vi "标样核查.vi"(11 "标样核查配置":T1={"数据保存间隔"=1.0, "水温标样值"=0.0, "pH标样值"=0.0, "溶解氧标样值"=0.0, "电导率标样值"=0.0, "浊度标样值"=0.0}) -> ()   [LabVIEW 2016, in "斯坦道多参数.lvlib"]
panel:
  out "运行状态":u16(ring) items=["空闲", "水样测试", "标样核查"]
  out "seconds since 1Jan1904":timestamp
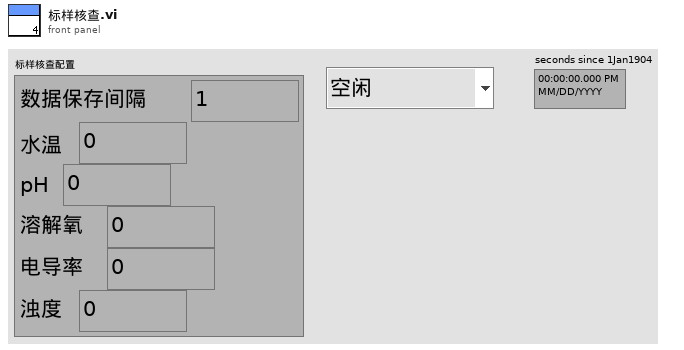
[diagram p1: front panel]
types:
  T1 = cluster{"数据保存间隔":dbl, "水温标样值":dbl, "pH标样值":dbl, "溶解氧标样值":dbl, "电导率标样值":dbl, "浊度标样值":dbl}
  T2 = cluster{"因子编码":string, "单位":string, "标样参考值":sgl, "水样数据时间":timestamp, "水样实测值":sgl, "水样数据标识":string, "探头温度":sgl}
  T3 = typedef "LVDateTimeRec.ctl" = cluster{"秒数的小数部分":dbl, "秒":i32, "分":i32, "时":i32, "日":i32, "月":i32, "年":i32, "天数（周）":i32, "天数（年）":i32, "DST":i32}
  T4 = cluster{"温度测量值":sgl, "DO%":sgl, "DOmg/L":sgl, "温度偏移修正值":sgl}
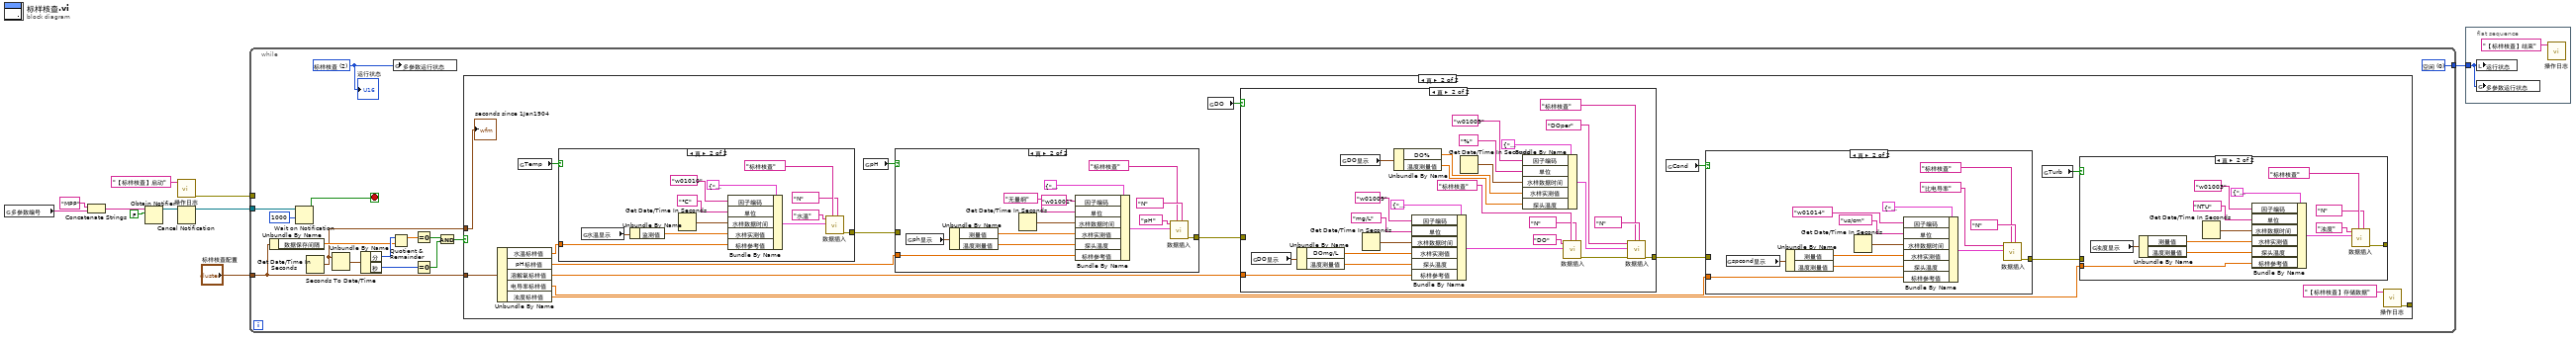
[diagram p0: block diagram]
diagram:
  n1 = global read "多参数全局变量.vi" "多参数编号"() -> (w3:string)
  n2 = Concatenate Strings("MPP" ("名称（未命名）"), w3) -> (w4:string)
  n3 = Obtain Notifier(name (unnamed)=w4, notification data type=FALSE) -> (notifier out=w7:refnum<notifier>)  [unwired: 2 in, 2 out]
  n4 = call "操作日志.vi"("日志信息"="【标样核查】启动") -> ("error out"=w1:errorcluster)  [unwired: 10 in]
  n5 = Cancel Notification(0:w7) -> (8:w6:refnum<notifier>)  [unwired: 1 in, 2 out]
  n6 = while {
    tunnel: "标样核查配置" -> [w21]
    tunnel: [w15] -> w5
    tunnel: w6 -> [w14]
    tunnel: w1 -> [_]
    stop <- w12 stop-if-true
    w15 = u16 0 items=["空闲", "水样测试", "标样核查"] ("多参数运行状态")
    w11 = u16 2 items=["空闲", "水样测试", "标样核查"] ("多参数运行状态")
    n7 = Unbundle By Name(w21) -> ("数据保存间隔"=w19:dbl)
    n8 = Wait on Notification(notifier=w14, timeout in ms (-1)=1000 ("超时毫秒(-1)")) -> (notification=w12:bool)  [unwired: 2 in, 3 out]
    n9 = Get Date/Time In Seconds() -> (seconds since 1Jan1904=w16:timestamp)
    n10 = Seconds To Date/Time(time stamp (now)=w16) -> (date time rec=w25:T3)  [unwired: 1 in]
    n11 = Unbundle By Name(w25) -> ("分"=w20:i32, "秒"=w24:i32)
    n12 = Quotient & Remainder(x=w20, y=w19) -> (x-y*floor(x/y)=w18:dbl)  [unwired: 1 out]
    n13 = global write "多参数全局变量.vi" "多参数运行状态"(w11) -> ()
    n14 = Equal To 0?(x=w18) -> (x = 0?=w17:bool)
    n15 = Equal To 0?(x=w24) -> (x = 0?=w23:bool)
    n16 = And(x=w17, y=w23) -> (x .and. y?=w22:bool)
    n17 = case shown="真" w22 {
      tunnel: w21 -> [_ w33]
      tunnel: w16 -> [_ w43]
      tunnel: [_ w26] -> _
      frame False {
      }
      frame True {
        n18 = Unbundle By Name(w33) -> ("水温标样值"=w32:dbl, "pH标样值"=w31:dbl, "溶解氧标样值"=w30:dbl, "电导率标样值"=w29:dbl, "浊度标样值"=w28:dbl)
        n19 = global read "断电保存变量.vi" "Temp"() -> (w38:bool)
        n20 = case shown="真" w38 {
          tunnel: [_ w111] -> w42
          tunnel: w32 -> [_ w110]
          frame False {
          }
          frame True {
            n21 = global read "多参数全局变量.vi" "水温显示"() -> (w109:cluster{"CH":u16, "监测值":dbl, "温度偏移修正值":sgl})
            n22 = Unbundle By Name(w109) -> ("监测值"=w108:dbl)
            n23 = Get Date/Time In Seconds() -> (seconds since 1Jan1904=w118:timestamp)
            n24 = Bundle By Name(cluster=T2 {"因子编码"="w01003", "单位"="无量纲", "标样参考值"=0.0, "水样数据时间"=timestamp(0 s since 1904-01-01), "水样实测值"=0.0, "水样数据标识"="N", "探头温度"=0.0} ("data in"), "因子编码"="w01010", "单位"="℃", "水样数据时间"=w118, "水样实测值"=w108, "标样参考值"=w110) -> (w117:T2)
            n25 = call "数据插入.vi"("数据标记表"="N", "测量模式"="标样核查", "data in"=w117, "table输入"="水温") -> ("error out"=w111:errorcluster)  [unwired: 7 in]
          }
        }
        n26 = global read "断电保存变量.vi" "pH"() -> (w37:bool)
        n27 = case shown="真" w37 {
          tunnel: w42 -> [_ _]
          tunnel: [_ w99] -> w41
          tunnel: w31 -> [_ w98]
          frame False {
          }
          frame True {
            n28 = global read "多参数全局变量.vi" "ph显示"() -> (w97:cluster{"温度测量值":sgl, "测量值":sgl, "温度偏移修正值":sgl})
            n29 = Unbundle By Name(w97) -> ("测量值"=w96:sgl, "温度测量值"=w95:sgl)
            n30 = Get Date/Time In Seconds() -> (seconds since 1Jan1904=w104:timestamp)
            n31 = Bundle By Name(cluster=T2 {"因子编码"="w01003", "单位"="无量纲", "标样参考值"=0.0, "水样数据时间"=timestamp(0 s since 1904-01-01), "水样实测值"=0.0, "水样数据标识"="N", "探头温度"=0.0} ("data in"), "因子编码"="w01001", "单位"="无量纲", "水样数据时间"=w104, "水样实测值"=w96, "探头温度"=w95, "标样参考值"=w98) -> (w105:T2)
            n32 = call "数据插入.vi"("数据标记表"="N", "测量模式"="标样核查", "data in"=w105, "table输入"="pH") -> ("error out"=w99:errorcluster)  [unwired: 7 in]
          }
        }
        n33 = global read "断电保存变量.vi" "DO"() -> (w36:bool)
        n34 = case shown="真" w36 {
          tunnel: w41 -> [_ _]
          tunnel: [_ w82] -> w40
          tunnel: w30 -> [_ w84]
          frame False {
          }
          frame True {
            n35 = global read "多参数全局变量.vi" "DO显示"() -> (w70:T4)
            n36 = Unbundle By Name(w70) -> ("DOmg/L"=w92:sgl, "温度测量值"=w94:sgl)
            n37 = global read "多参数全局变量.vi" "DO显示"() -> (w71:T4)
            n38 = Get Date/Time In Seconds() -> (seconds since 1Jan1904=w91:timestamp)
            n39 = Unbundle By Name(w71) -> ("DO%"=w75:sgl, "温度测量值"=w73:sgl)
            n40 = Bundle By Name(cluster=T2 {"因子编码"="w01003", "单位"="无量纲", "标样参考值"=0.0, "水样数据时间"=timestamp(0 s since 1904-01-01), "水样实测值"=0.0, "水样数据标识"="N", "探头温度"=0.0} ("data in"), "因子编码"="w01009", "单位"="mg/L", "水样数据时间"=w91, "水样实测值"=w92, "探头温度"=w94, "标样参考值"=w84) -> (w90:T2)
            n41 = Get Date/Time In Seconds() -> (seconds since 1Jan1904=w76:timestamp)
            n42 = Bundle By Name(cluster=T2 {"因子编码"="w01003", "单位"="无量纲", "标样参考值"=0.0, "水样数据时间"=timestamp(0 s since 1904-01-01), "水样实测值"=0.0, "水样数据标识"="N", "探头温度"=0.0} ("data in"), "因子编码"="w01009", "单位"="%", "水样数据时间"=w76, "水样实测值"=w75, "探头温度"=w73) -> (w72:T2)
            n43 = call "数据插入.vi"("数据标记表"="N", "测量模式"="标样核查", "data in"=w90, "table输入"="DO") -> ("error out"=w83:errorcluster)  [unwired: 7 in]
            n44 = call "数据插入.vi"("数据标记表"="N", "测量模式"="标样核查", "error in (no error)"=w83, "data in"=w72, "table输入"="DOper") -> ("error out"=w82:errorcluster)  [unwired: 6 in]
          }
        }
        n45 = global read "断电保存变量.vi" "Cond"() -> (w35:bool)
        n46 = case shown="真" w35 {
          tunnel: w40 -> [_ _]
          tunnel: [_ w61] -> w39
          tunnel: w29 -> [_ w60]
          frame False {
          }
          frame True {
            n47 = global read "多参数全局变量.vi" "spcond显示"() -> (w59:cluster{"温度测量值":sgl, "测量值":sgl, "温度偏移修正值":sgl})
            n48 = Unbundle By Name(w59) -> ("测量值"=w58:sgl, "温度测量值"=w57:sgl)
            n49 = Get Date/Time In Seconds() -> (seconds since 1Jan1904=w66:timestamp)
            n50 = Bundle By Name(cluster=T2 {"因子编码"="w01003", "单位"="无量纲", "标样参考值"=0.0, "水样数据时间"=timestamp(0 s since 1904-01-01), "水样实测值"=0.0, "水样数据标识"="N", "探头温度"=0.0} ("data in"), "因子编码"="w01014", "单位"="us/cm", "水样数据时间"=w66, "水样实测值"=w58, "探头温度"=w57, "标样参考值"=w60) -> (w67:T2)
            n51 = call "数据插入.vi"("数据标记表"="N", "测量模式"="标样核查", "data in"=w67, "table输入"="比电导率") -> ("error out"=w61:errorcluster)  [unwired: 7 in]
          }
        }
        n52 = global read "断电保存变量.vi" "Turb"() -> (w34:bool)
        n53 = case shown="真" w34 {
          tunnel: w39 -> [_ _]
          tunnel: [_ w48] -> _
          tunnel: w28 -> [_ w47]
          frame False {
          }
          frame True {
            n54 = global read "多参数全局变量.vi" "浊度显示"() -> (w46:cluster{"温度测量值":sgl, "测量值":sgl, "温度偏移修正值":sgl})
            n55 = Unbundle By Name(w46) -> ("测量值"=w45:sgl, "温度测量值"=w44:sgl)
            n56 = Get Date/Time In Seconds() -> (seconds since 1Jan1904=w55:timestamp)
            n57 = Bundle By Name(cluster=T2 {"因子编码"="w01003", "单位"="无量纲", "标样参考值"=0.0, "水样数据时间"=timestamp(0 s since 1904-01-01), "水样实测值"=0.0, "水样数据标识"="N", "探头温度"=0.0} ("data in"), "因子编码"="w01003", "单位"="NTU", "水样数据时间"=w55, "水样实测值"=w45, "探头温度"=w44, "标样参考值"=w47) -> (w54:T2)
            n58 = call "数据插入.vi"("数据标记表"="N", "测量模式"="标样核查", "data in"=w54, "table输入"="浊度") -> ("error out"=w48:errorcluster)  [unwired: 7 in]
          }
        }
        n59 = call "操作日志.vi"("日志信息"="【标样核查】存储数据") -> ("error out"=w26:errorcluster)  [unwired: 10 in]
        "seconds since 1Jan1904" <- w43
      }
    }
    "运行状态" <- w11
  }
  n60 = flat-sequence {
    tunnel: w5 -> [w121]
    frame #0 {
      n61 = local write "运行状态"(w121) -> ()
      n62 = global write "多参数全局变量.vi" "多参数运行状态"(w121) -> ()
      n63 = call "操作日志.vi"("日志信息"="【标样核查】结束") -> ()  [unwired: 10 in, 1 out]
    }
  }
